vi "DDAQ-Load-Keywords.vi"(11 "Path to Keywords CSV":path) -> (3 "Diodes Keywords Array":T1[](array[typedef]))   [LabVIEW 2020]
uses:
  DDAQ-Keyword.ctl
  <vilib>/Utility/file.llb/Read Delimited Spreadsheet (string).vi
panel:
  out "Array":string[](array[string])
  out "subarray 2":string[][](array[string])
  out "subarray":string[](array[string])
  out "all rows":string[][](array[string])
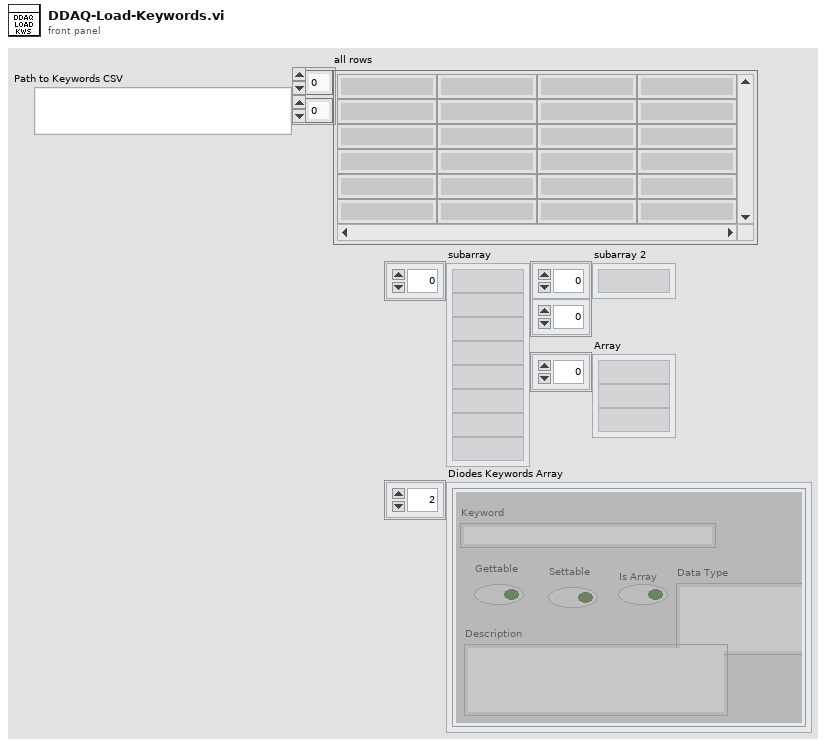
[diagram p1: front panel]
types:
  T1 = typedef "DDAQ-Keyword.ctl" = cluster{"Keyword":string, "Gettable":bool, "Settable":bool, "Is Array":bool, "Data Type":string, "Description":string}
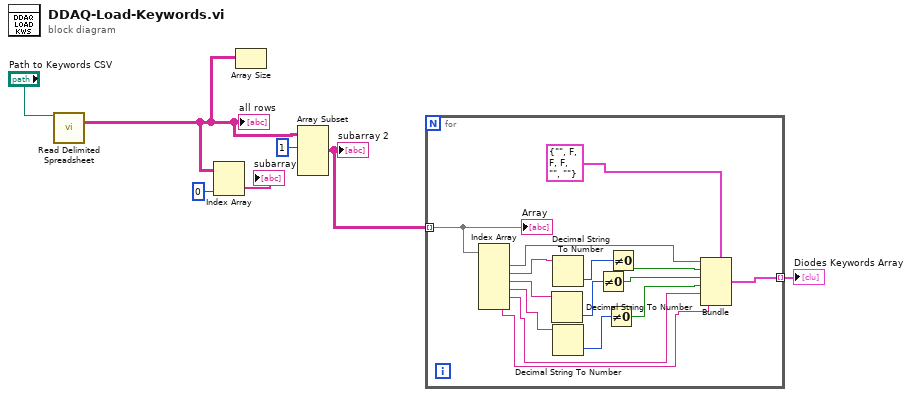
[diagram p0: block diagram]
diagram:
  n1 = call-poly <vilib>:"Read Delimited Spreadsheet.vi"("file path (dialog if empty)"="Path to Keywords CSV") -> ("all rows"=w5:string[][])  [unwired: 9 in, 5 out]
  "all rows" <- w5
  n2 = Index Array(array=w5, index (col)=0 ("disabled index (col)")) -> (element=→"subarray":string[])  [unwired: 1 in]
  n3 = Array Size(array=w5) -> ()  [unwired: 1 out]
  n4 = Array Subset(array=w5, index (row)=1 ("index")) -> (w3:string[][])  [unwired: 3 in]
  "subarray 2" <- w3
  n5 = for {
    tunnel: w3 -> [w22] mode=indexing
    tunnel: [w15] -> w2 mode=indexing
    n6 = Index Array(array=w22) -> (element #1=w12:string, element #2=w11:string, element #3=w16:string, element #4=w10:string, element #5=w13:string, element #6=w14:string)  [unwired: 6 in]
    n7 = Decimal String To Number(string=w16) -> (number=w18:i32)  [unwired: 2 in, 1 out]
    n8 = Decimal String To Number(string=w11) -> (number=w20:i32)  [unwired: 2 in, 1 out]
    n9 = Decimal String To Number(string=w10) -> (number=w9:i32)  [unwired: 2 in, 1 out]
    n10 = Not Equal To 0?(x=w18) -> (x != 0?=w17:bool)
    n11 = Not Equal To 0?(x=w9) -> (x != 0?=w8:bool)
    n12 = Not Equal To 0?(x=w20) -> (x != 0?=w19:bool)
    n13 = Bundle(cluster=T1 {"Keyword"="", "Gettable"=FALSE, "Settable"=FALSE, "Is Array"=FALSE, "Data Type"="", "Description"=""} ("Diode Keyword"), "Keyword"=w12, "Gettable"=w19, "Settable"=w17, "Is Array"=w8, "Data Type"=w13, "Description"=w14) -> (w15:T1)
    "Array" <- w22
  }
  "Diodes Keywords Array" <- w2
